vi "ControlPanelPeriodic.vi"() -> ()   [LabVIEW 2019]
uses:
  <vilib>/Utility/config.llb/NI_LVConfig.lvlib
  <vilib>/Utility/config.llb/Read Key (Double).vi
panel:
  out "TRUE 3":bool
  out "Loop Count 2":i32
  out "Numeric 2":i32
  out "Scaler":i8=127
  out "Color Match Name":string
  out "Normalized Color 2":cluster{"R":dbl, "G":dbl, "B":dbl}
  out "element 3":bool
  out "Color is matched":bool
  out "element 2":bool
  out "element":bool
  out "TRUE 2":bool
  out "TRUE 1":bool
  out "Loop Count":i32
  out "Numeric":i32
  out "Matched Color Name":string
  out "Confidence":dbl
  out "Matched Color":cluster{"R":dbl, "G":dbl, "B":dbl}
  out "Color":u32(colorbox)
  out "Normalized Color":cluster{"R":dbl, "G":dbl, "B":dbl}
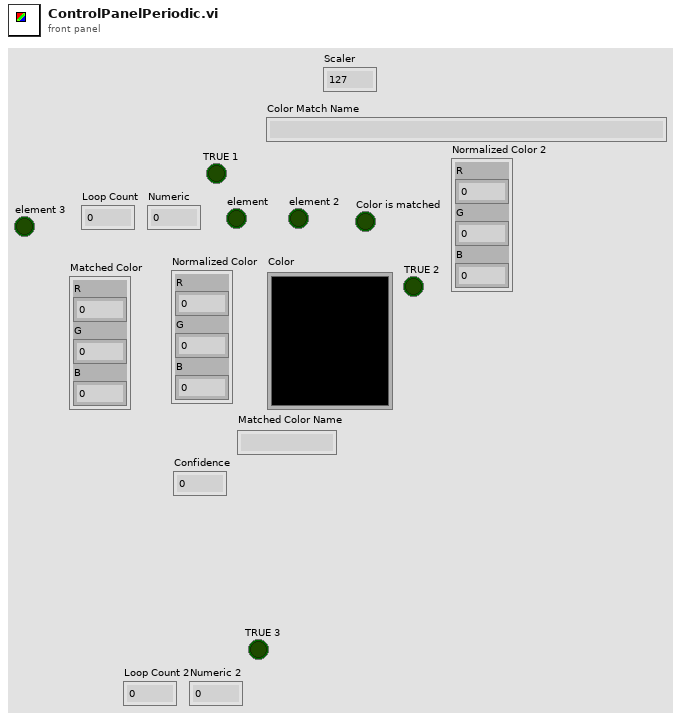
[diagram p1: front panel]
types:
  T1 = typedef "NI_LVConfig.lvlib/Config Data RefNum.ctl" = refnum<k1>
  T2 = typedef "WPI_JoystickDevRef.ctl" = cluster{"Device":T3}
  T3 = typedef "WPI_JoystickDeviceEnum.ctl" = enum16{"USB 0", "USB 1", "USB 2", "USB 3", "USB 4", "USB 5"}
  T4 = typedef "Color Sensor V3 DevRef.ctl" = cluster{"I2CDevRef":T5}
  T5 = typedef "WPI_I2CDevRef.ctl" = cluster{"DevStatus":errorcluster, "Device Address":u8, "Handle":i32, "I2C Bus":T6}
  T6 = typedef "i2c_bus.ctl" = enum16{"I2C On-Board", "I2C MXP", "Invalid"}
  T7 = typedef "WPI_MotorControlDeviceRef.ctl" = cluster{"DeviceStatus":errorcluster, "Type":T8, "PWM":cluster{"PWM Channel":T9, "DeadBand":T10}, "CAN":cluster{"Device Number":u8, "SetOutput VI Ref":variant, "GetOutput VI Ref":variant, "Enable VI Ref":variant, "Disable VI Ref":variant, "Data":variant}, "Invert":bool, "DIO PWM":cluster{"PWM \"Enable\" Channel":T9, "DIOChannel":T11, "PWM Rate":dbl}}
  T8 = typedef "WPI_MotorControlType.ctl" = enum16{"PWM", "CAN", "DIO PWM"}
  T9 = typedef "FPGA_DIOPWMChannel.ctl" = enum8{"PWM 0", "PWM 1", "PWM 2", "PWM 3", "PWM 4", "PWM 5", "PWM 6", "PWM 7", "PWM 8", "PWM 9", "PWM MXP 0", "PWM MXP 1", "PWM MXP 2", "PWM MXP 3", "PWM MXP 4", "PWM MXP 5", "PWM MXP 6", "PWM MXP 7", "PWM MXP 8", "PWM MXP 9", "Invalid"}
  T10 = typedef "WPI_PWMDeadband.ctl" = cluster{"Name":string, "maxPositivePwm":i32, "minPositivePwm":i32, "centerPwm":i32, "maxNegativePwm":i32, "minNegativePwm":i32, "angularRange":u16}
  T11 = typedef "FPGA_DIOChannel.ctl" = enum8{"DIO 0", "DIO 1", "DIO 2", "DIO 3", "DIO 4", "DIO 5", "DIO 6", "DIO 7", "DIO 8", "DIO 9", "DIO MXP 0", "DIO MXP 1", "DIO MXP 2", "DIO MXP 3", "DIO MXP 4", "DIO MXP 5", "DIO MXP 6", "DIO MXP 7", "DIO MXP 8", "DIO MXP 9", "DIO MXP 10", "DIO MXP 11", "DIO MXP 12", "DIO MXP 13", "DIO MXP 14", "DIO MXP 15", "SPI Port CS1", "SPI Port CS2", "SPI Port CS3", "SPI Port MISO", "SPI Port MOSI", "Invalid"}
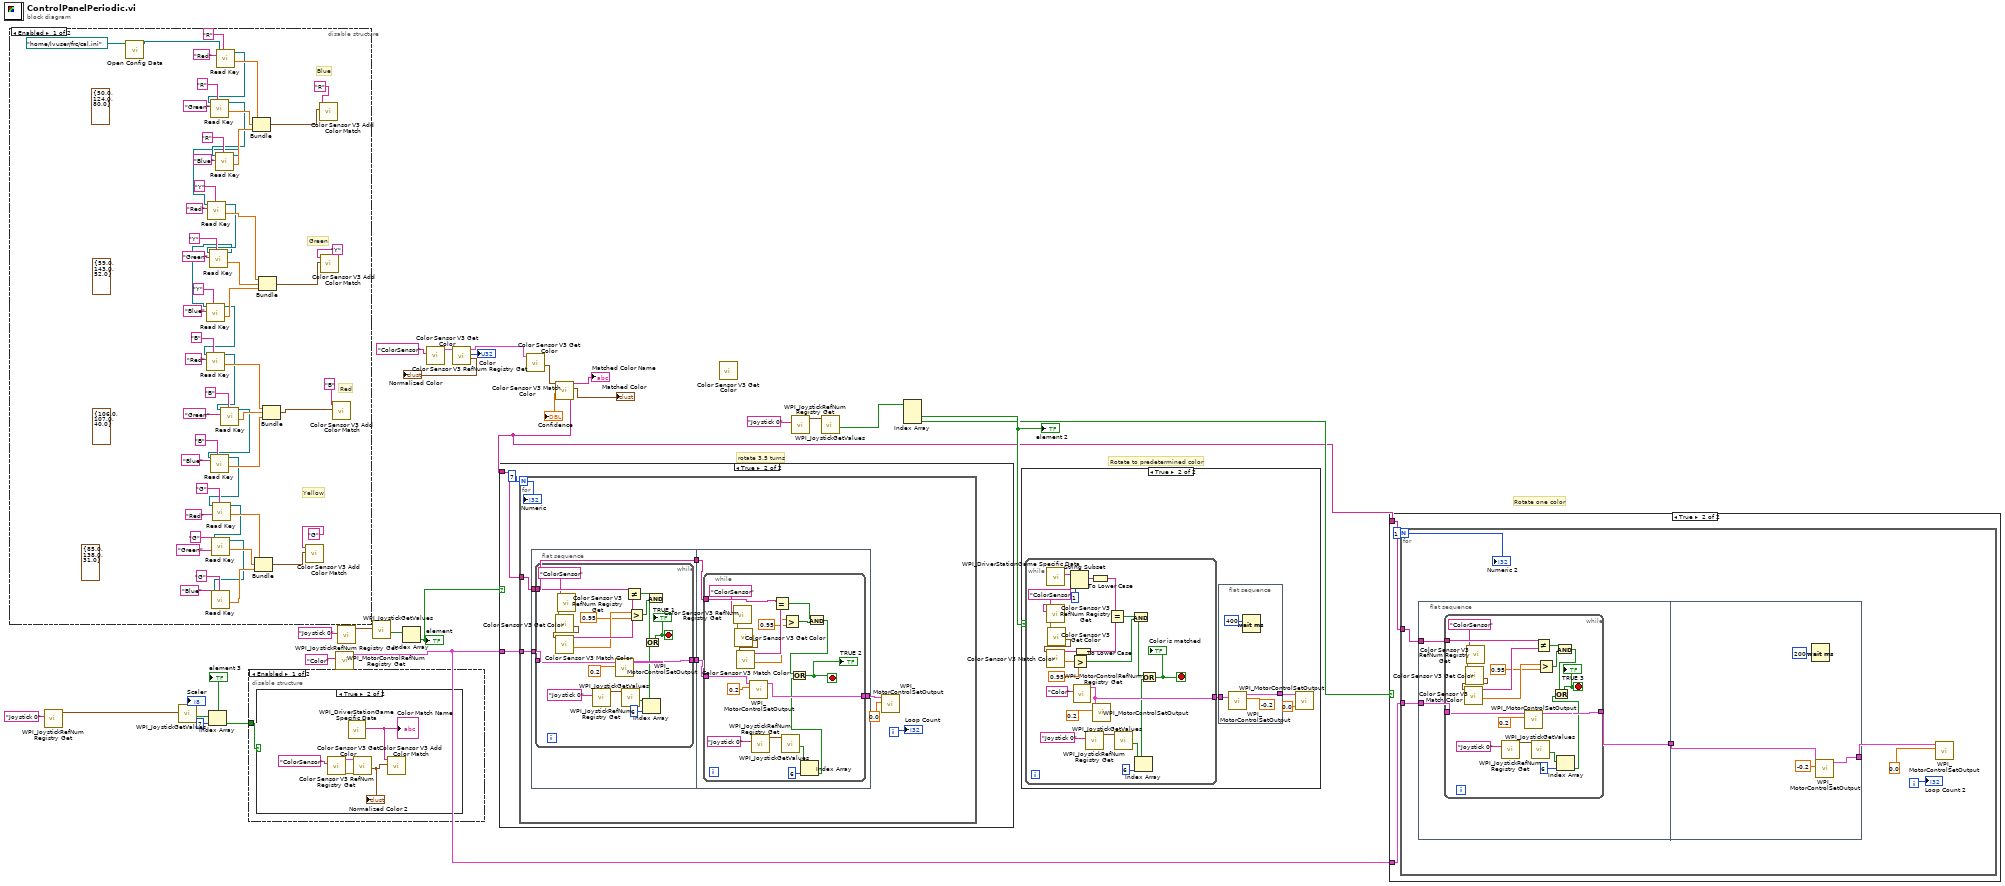
[diagram p0: block diagram]
diagram:
  # "rotate 3.5 turns"
  # "Rotate to predetermined color"
  # "Rotate one color"
  n1 = disable-structure shown="Enabled" {
    frame Enabled {
      (unwired) cluster{"R":dbl, "G":dbl, "B":dbl} {"R"=85.0, "G"=138.0, "B"=31.0} ("Color")
      (unwired) cluster{"R":dbl, "G":dbl, "B":dbl} {"R"=106.0, "G"=107.0, "B"=40.0} ("Color")
      (unwired) cluster{"R":dbl, "G":dbl, "B":dbl} {"R"=59.0, "G"=143.0, "B"=52.0} ("Color")
      (unwired) cluster{"R":dbl, "G":dbl, "B":dbl} {"R"=50.0, "G"=124.0, "B"=80.0} ("Color")
      # "Red"
      # "Green"
      # "Yellow"
      # "Blue"
      n2 = call <vilib>:"Open Config Data.vi"("configuration file path"=path "/home/lvuser/frc/cal.ini") -> ("refnum"=w27:T1)  [unwired: 8 in, 2 out]
      n3 = call-poly <vilib>:"Read Key.vi"("section"="R", "key"="Red", "refnum"=w27) -> ("value"=w52:dbl, "refnum out"=w51:T1)  [unwired: 5 in, 2 out]
      n4 = call-poly <vilib>:"Read Key.vi"("section"="R", "key"="Green", "refnum"=w51) -> ("value"=w53:dbl, "refnum out"=w50:T1)  [unwired: 5 in, 2 out]
      n5 = call-poly <vilib>:"Read Key.vi"("section"="R", "key"="Blue", "refnum"=w50) -> ("value"=w54:dbl, "refnum out"=w49:T1)  [unwired: 5 in, 2 out]
      n6 = call-poly <vilib>:"Read Key.vi"("section"="Y", "key"="Red", "refnum"=w49) -> ("value"=w48:dbl, "refnum out"=w35:T1)  [unwired: 5 in, 2 out]
      n7 = call-poly <vilib>:"Read Key.vi"("section"="Y", "key"="Green", "refnum"=w35) -> ("value"=w47:dbl, "refnum out"=w34:T1)  [unwired: 5 in, 2 out]
      n8 = call-poly <vilib>:"Read Key.vi"("section"="Y", "key"="Blue", "refnum"=w34) -> ("value"=w46:dbl, "refnum out"=w33:T1)  [unwired: 5 in, 2 out]
      n9 = call-poly <vilib>:"Read Key.vi"("section"="B", "key"="Red", "refnum"=w33) -> ("value"=w40:dbl, "refnum out"=w32:T1)  [unwired: 5 in, 2 out]
      n10 = call-poly <vilib>:"Read Key.vi"("section"="B", "key"="Green", "refnum"=w32) -> ("value"=w42:dbl, "refnum out"=w31:T1)  [unwired: 5 in, 2 out]
      n11 = call-poly <vilib>:"Read Key.vi"("section"="B", "key"="Blue", "refnum"=w31) -> ("value"=w41:dbl, "refnum out"=w30:T1)  [unwired: 5 in, 2 out]
      n12 = call-poly <vilib>:"Read Key.vi"("section"="G", "key"="Red", "refnum"=w30) -> ("value"=w43:dbl, "refnum out"=w29:T1)  [unwired: 5 in, 2 out]
      n13 = call-poly <vilib>:"Read Key.vi"("section"="G", "key"="Green", "refnum"=w29) -> ("value"=w44:dbl, "refnum out"=w28:T1)  [unwired: 5 in, 2 out]
      n14 = call-poly <vilib>:"Read Key.vi"("section"="G", "key"="Blue", "refnum"=w28) -> ("value"=w45:dbl)  [unwired: 5 in, 3 out]
      n15 = Bundle("value"=w52, "value"=w53, "value"=w54) -> (w36:cluster{"value":dbl, "value":dbl, "value":dbl})  [unwired: 1 in]
      n16 = Bundle("value"=w43, "value"=w44, "value"=w45) -> (w38:cluster{"value":dbl, "value":dbl, "value":dbl})  [unwired: 1 in]
      n17 = Bundle("value"=w48, "value"=w47, "value"=w46) -> (w37:cluster{"value":dbl, "value":dbl, "value":dbl})  [unwired: 1 in]
      n18 = Bundle("value"=w40, "value"=w42, "value"=w41) -> (w39:cluster{"value":dbl, "value":dbl, "value":dbl})  [unwired: 1 in]
      n19 = call <vilib>:"Color Sensor V3 Add Color Match.vi"("Color"=w38, "Name"="G") -> ()  [unwired: 10 in]
      n20 = call <vilib>:"Color Sensor V3 Add Color Match.vi"("Color"=w36, "Name"="R") -> ()  [unwired: 10 in]
      n21 = call <vilib>:"Color Sensor V3 Add Color Match.vi"("Color"=w37, "Name"="Y") -> ()  [unwired: 10 in]
      n22 = call <vilib>:"Color Sensor V3 Add Color Match.vi"("Color"=w39, "Name"="B") -> ()  [unwired: 10 in]
    }
    frame Disabled {
    }
  }
  n23 = call <vilib>:"WPI_JoystickRefNum Registry Get.vi"("refnum name"="Joystick 0") -> ("JoystickDevRef"=w8:T2)  [unwired: 9 in, 1 out]
  n24 = call <vilib>:"WPI_JoystickGetValues.vi"("JoystickDevRef"=w8) -> ("Buttons"=w10:bool[])  [unwired: 6 in, 4 out]
  n25 = Index Array(array=w10, index=7) -> (element=w7:bool)
  "element 3" <- w7
  n26 = disable-structure shown="Enabled" {
    disable-tunnel: w7 -> [w83 _]
    frame Enabled {
      n27 = case shown="True" w83 {
        frame False {
        }
        frame True {
          n28 = call <vilib>:"Color Sensor V3 RefNum Registry Get.vi"("refnum name"="ColorSensor") -> ("error out"=w87:errorcluster, "ColorSensorDevRef"=w85:T4)  [unwired: 9 in]
          n29 = call <vilib>:"WPI_DriverStationGame Specific Data.vi"() -> ("Game Specific Data"=w88:string)  [unwired: 11 in]
          "Color Match Name" <- w88
          n30 = call <vilib>:"Color Sensor V3 Get Color.vi"("error in (no error)"=w87, "ColorSensorDevRef"=w85) -> ("Normalized Color"=w86:cluster{"R":dbl, "G":dbl, "B":dbl})  [unwired: 6 in, 3 out]
          "Normalized Color 2" <- w86
          n31 = call <vilib>:"Color Sensor V3 Add Color Match.vi"("Color"=w86, "Name"=w88) -> ()  [unwired: 10 in]
        }
      }
    }
    frame Disabled {
    }
  }
  n32 = call <vilib>:"WPI_MotorControlRefNum Registry Get.vi"("refnum name"="Color") -> ("MotorControlDevRef"=w2:T7)  [unwired: 9 in, 1 out]
  n33 = call <vilib>:"WPI_JoystickRefNum Registry Get.vi"("refnum name"="Joystick 0") -> ("JoystickDevRef"=w18:T2)  [unwired: 9 in, 1 out]
  n34 = call <vilib>:"WPI_JoystickGetValues.vi"("JoystickDevRef"=w18) -> ("Buttons"=w17:bool[])  [unwired: 6 in, 4 out]
  n35 = Index Array(array=w17) -> (element=w12:bool)  [unwired: 1 in]
  "element" <- w12
  n36 = call <vilib>:"Color Sensor V3 RefNum Registry Get.vi"("refnum name"="ColorSensor") -> ("ColorSensorDevRef"=w25:T4)  [unwired: 9 in, 1 out]
  n37 = call <vilib>:"Color Sensor V3 Get Color.vi"("ColorSensorDevRef"=w25) -> ("Normalized Color"=→"Normalized Color":cluster{"R":dbl, "G":dbl, "B":dbl}, "Color"=→"Color":u32, "ColorSensorDevRef out"=w4:T4)  [unwired: 7 in, 1 out]
  n38 = call <vilib>:"Color Sensor V3 Get Color.vi"("ColorSensorDevRef"=w4) -> ("Normalized Color"=w20:cluster{"R":dbl, "G":dbl, "B":dbl})  [unwired: 7 in, 3 out]
  n39 = call <vilib>:"Color Sensor V3 Match Color.vi"("Measured Color"=w20) -> ("Confidence"=→"Confidence":dbl, "Matched Color"=→"Matched Color":cluster{"R":dbl, "G":dbl, "B":dbl}, "Matched Color Name"=w1:string)  [unwired: 8 in]
  "Matched Color Name" <- w1
  n40 = case shown="True" w12 {
    tunnel: w1 -> [_ w91]
    tunnel: w2 -> [_ w90]
    frame False {
    }
    frame True {
      n41 = for {
        N: 7 -> [w94]
        tunnel: w91 -> [w97]
        tunnel: w90 -> [w96]
        i -> [w95]
        n42 = flat-sequence {
          tunnel: [w101] -> _
          tunnel: w97 -> [w101]
          tunnel: w96 -> [w102]
          tunnel: [w100] -> w99
          tunnel: [w101] -> w98
          tunnel: w99 -> [w124]
          tunnel: w98 -> [w125]
          tunnel: [w123] -> w92
          frame #0 {
            n43 = while {
              tunnel: w101 -> [w119]
              tunnel: w102 -> [w122]
              tunnel: [w111] -> w100
              stop <- w107 stop-if-true
              n44 = call <vilib>:"Color Sensor V3 RefNum Registry Get.vi"("refnum name"="ColorSensor") -> ("error out"=w118:errorcluster, "ColorSensorDevRef"=w117:T4)  [unwired: 9 in]
              n45 = call <vilib>:"Color Sensor V3 Get Color.vi"("error in (no error)"=w118, "ColorSensorDevRef"=w117) -> ("Normalized Color"=w116:cluster{"R":dbl, "G":dbl, "B":dbl})  [unwired: 6 in, 3 out]
              n46 = call <vilib>:"Color Sensor V3 Match Color.vi"("Measured Color"=w116) -> ("Confidence"=w114:dbl, "Matched Color Name"=w121:string)  [unwired: 8 in, 1 out]
              n47 = call <vilib>:"WPI_JoystickRefNum Registry Get.vi"("refnum name"="Joystick 0") -> ("JoystickDevRef"=w109:T2)  [unwired: 9 in, 1 out]
              n48 = call <vilib>:"WPI_MotorControlSetOutput.vi"("Output"=0.2 ("Motor Output"), "MotorControlDevRef"=w122) -> ("MotorControlDevRef"=w111:T7)  [unwired: 7 in, 2 out]
              n49 = call <vilib>:"WPI_JoystickGetValues.vi"("JoystickDevRef"=w109) -> ("Buttons"=w108:bool[])  [unwired: 6 in, 4 out]
              n50 = Not Equal?(x=w119, y=w121) -> (x != y?=w115:bool)
              n51 = Greater?(x=w114, y=0.95) -> (0:w112:bool)
              n52 = Index Array(array=w108, index=6) -> (element=w106:bool)
              n53 = And(x=w115, y=w112) -> (x .and. y?=w105:bool)
              n54 = Or(x=w105, y=w106) -> (x .or. y?=w107:bool)
              "TRUE 1" <- w107
            }
          }
          frame #1 {
            n55 = while {
              tunnel: w125 -> [w143]
              tunnel: w124 -> [w145]
              tunnel: [w134] -> w123
              stop <- w128 stop-if-true
              n56 = call <vilib>:"Color Sensor V3 RefNum Registry Get.vi"("refnum name"="ColorSensor") -> ("error out"=w142:errorcluster, "ColorSensorDevRef"=w141:T4)  [unwired: 9 in]
              n57 = call <vilib>:"Color Sensor V3 Get Color.vi"("error in (no error)"=w142, "ColorSensorDevRef"=w141) -> ("Normalized Color"=w140:cluster{"R":dbl, "G":dbl, "B":dbl})  [unwired: 6 in, 3 out]
              n58 = call <vilib>:"Color Sensor V3 Match Color.vi"("Measured Color"=w140) -> ("Confidence"=w136:dbl, "Matched Color Name"=w144:string)  [unwired: 8 in, 1 out]
              n59 = call <vilib>:"WPI_MotorControlSetOutput.vi"("Output"=0.2, "MotorControlDevRef"=w145) -> ("MotorControlDevRef"=w134:T7)  [unwired: 7 in, 2 out]
              n60 = call <vilib>:"WPI_JoystickRefNum Registry Get.vi"("refnum name"="Joystick 0") -> ("JoystickDevRef"=w132:T2)  [unwired: 9 in, 1 out]
              n61 = Equal?(x=w143, y=w144) -> (x = y?=w137:bool)
              n62 = call <vilib>:"WPI_JoystickGetValues.vi"("JoystickDevRef"=w132) -> ("Buttons"=w131:bool[])  [unwired: 6 in, 4 out]
              n63 = Greater?(x=w136, y=0.95) -> (0:w138:bool)
              n64 = Index Array(array=w131, index=6) -> (element=w130:bool)
              n65 = And(x=w137, y=w138) -> (x .and. y?=w129:bool)
              n66 = Or(x=w129, y=w130) -> (x .or. y?=w128:bool)
              "TRUE 2" <- w128
            }
          }
        }
        n67 = call <vilib>:"WPI_MotorControlSetOutput.vi"("Output"=0.0, "MotorControlDevRef"=w92) -> ()  [unwired: 7 in, 3 out]
        "Loop Count" <- w95
        "Numeric" <- w94
      }
    }
  }
  n68 = call <vilib>:"Color Sensor V3 Get Color.vi"() -> ()  [unwired: 8 in, 4 out]
  n69 = call <vilib>:"WPI_JoystickRefNum Registry Get.vi"("refnum name"="Joystick 0") -> ("JoystickDevRef"=w15:T2)  [unwired: 9 in, 1 out]
  n70 = call <vilib>:"WPI_JoystickGetValues.vi"("JoystickDevRef"=w15) -> ("Buttons"=w14:bool[])  [unwired: 6 in, 4 out]
  n71 = Index Array(array=w14) -> (element #2=w13:bool, element #3=w3:bool)  [unwired: 3 in, 1 out]
  "element 2" <- w13
  n72 = case shown="True" w13 {
    frame False {
    }
    frame True {
      n73 = while {
        tunnel: [w170] -> w147
        stop <- w155 stop-if-true
        n74 = call <vilib>:"Color Sensor V3 RefNum Registry Get.vi"("refnum name"="ColorSensor") -> ("error out"=w174:errorcluster, "ColorSensorDevRef"=w173:T4)  [unwired: 9 in]
        n75 = call <vilib>:"WPI_DriverStationGame Specific Data.vi"() -> ("Game Specific Data"=w165:string)  [unwired: 11 in]
        n76 = call <vilib>:"Color Sensor V3 Get Color.vi"("error in (no error)"=w174, "ColorSensorDevRef"=w173) -> ("Normalized Color"=w172:cluster{"R":dbl, "G":dbl, "B":dbl})  [unwired: 6 in, 3 out]
        n77 = call <vilib>:"Color Sensor V3 Match Color.vi"("Measured Color"=w172) -> ("Confidence"=w168:dbl, "Matched Color Name"=w176:string)  [unwired: 8 in, 1 out]
        n78 = String Subset(string=w165, length (rest)=1 ("length (rest)")) -> (substring=w162:string)  [unwired: 1 in]
        n79 = Greater?(x=w168, y=0.95) -> (0:w166:bool)
        n80 = call <vilib>:"WPI_MotorControlRefNum Registry Get.vi"("refnum name"="Color") -> ("MotorControlDevRef"=w170:T7)  [unwired: 9 in, 1 out]
        n81 = To Lower Case(string=w176) -> (all lower case string=w164:string)
        n82 = call <vilib>:"WPI_JoystickRefNum Registry Get.vi"("refnum name"="Joystick 0") -> ("JoystickDevRef"=w159:T2)  [unwired: 9 in, 1 out]
        n83 = To Lower Case(string=w162) -> (all lower case string=w163:string)
        n84 = call <vilib>:"WPI_MotorControlSetOutput.vi"("Output"=0.2 ("Motor Output"), "MotorControlDevRef"=w170) -> ()  [unwired: 7 in, 3 out]
        n85 = Equal?(x=w163, y=w164) -> (x = y?=w169:bool)
        n86 = call <vilib>:"WPI_JoystickGetValues.vi"("JoystickDevRef"=w159) -> ("Buttons"=w158:bool[])  [unwired: 6 in, 4 out]
        n87 = And(x=w169, y=w166) -> (x .and. y?=w156:bool)
        n88 = Index Array(array=w158, index=6) -> (element=w157:bool)
        n89 = Or(x=w156, y=w157) -> (x .or. y?=w155:bool)
        "Color is matched" <- w155
      }
      n90 = flat-sequence {
        tunnel: w147 -> [w152]
        tunnel: [w149] -> w146
        frame #0 {
          n91 = call <vilib>:"WPI_MotorControlSetOutput.vi"("Output"=-0.2, "MotorControlDevRef"=w152) -> ("MotorControlDevRef"=w149:T7)  [unwired: 7 in, 2 out]
          n92 = Wait (ms)(milliseconds to wait=u32 400) -> ()  [unwired: 1 out]
        }
      }
      n93 = call <vilib>:"WPI_MotorControlSetOutput.vi"("Output"=0.0, "MotorControlDevRef"=w146) -> ()  [unwired: 7 in, 3 out]
    }
  }
  n94 = case shown="True" w3 {
    tunnel: w2 -> [_ w178]
    tunnel: w1 -> [_ w177]
    frame False {
    }
    frame True {
      n95 = for {
        N: 1 -> [w183]
        tunnel: w177 -> [w186]
        tunnel: w178 -> [w185]
        i -> [w184]
        n96 = flat-sequence {
          tunnel: [w188] -> _
          tunnel: w186 -> [w188]
          tunnel: w185 -> [w189]
          tunnel: [w187] -> w181
          tunnel: w181 -> [w211]
          tunnel: [w210] -> w180
          frame #0 {
            n97 = while {
              tunnel: w188 -> [w206]
              tunnel: w189 -> [w209]
              tunnel: [w198] -> w187
              stop <- w194 stop-if-true
              n98 = call <vilib>:"Color Sensor V3 RefNum Registry Get.vi"("refnum name"="ColorSensor") -> ("error out"=w205:errorcluster, "ColorSensorDevRef"=w204:T4)  [unwired: 9 in]
              n99 = call <vilib>:"Color Sensor V3 Get Color.vi"("error in (no error)"=w205, "ColorSensorDevRef"=w204) -> ("Normalized Color"=w203:cluster{"R":dbl, "G":dbl, "B":dbl})  [unwired: 6 in, 3 out]
              n100 = call <vilib>:"Color Sensor V3 Match Color.vi"("Measured Color"=w203) -> ("Confidence"=w201:dbl, "Matched Color Name"=w208:string)  [unwired: 8 in, 1 out]
              n101 = call <vilib>:"WPI_JoystickRefNum Registry Get.vi"("refnum name"="Joystick 0") -> ("JoystickDevRef"=w196:T2)  [unwired: 9 in, 1 out]
              n102 = call <vilib>:"WPI_MotorControlSetOutput.vi"("Output"=0.2 ("Motor Output"), "MotorControlDevRef"=w209) -> ("MotorControlDevRef"=w198:T7)  [unwired: 7 in, 2 out]
              n103 = call <vilib>:"WPI_JoystickGetValues.vi"("JoystickDevRef"=w196) -> ("Buttons"=w195:bool[])  [unwired: 6 in, 4 out]
              n104 = Not Equal?(x=w206, y=w208) -> (x != y?=w202:bool)
              n105 = Greater?(x=w201, y=0.95) -> (0:w199:bool)
              n106 = And(x=w202, y=w199) -> (x .and. y?=w192:bool)
              n107 = Index Array(array=w195, index=6) -> (element=w193:bool)
              n108 = Or(x=w192, y=w193) -> (x .or. y?=w194:bool)
              "TRUE 3" <- w194
            }
          }
          frame #1 {
            n109 = Wait (ms)(milliseconds to wait=u32 200) -> ()  [unwired: 1 out]
            n110 = call <vilib>:"WPI_MotorControlSetOutput.vi"("Output"=-0.2, "MotorControlDevRef"=w211) -> ("MotorControlDevRef"=w210:T7)  [unwired: 7 in, 2 out]
          }
        }
        n111 = call <vilib>:"WPI_MotorControlSetOutput.vi"("Output"=0.0, "MotorControlDevRef"=w180) -> ()  [unwired: 7 in, 3 out]
        "Loop Count 2" <- w184
        "Numeric 2" <- w183
      }
    }
  }
